vi "Load Settings from XML.vi"(8 "error in (no error)":errorcluster, 11 "Settings in":T1) -> (0 "error out":errorcluster, 3 "Settings out":T1)   [LabVIEW 2019, in "Settings.lvlib"]
doc: "Attempts to load previous user specified settings from an XML file.\n\nThis VI will not generate an error. If a suitable XML file can't be loaded and parsed then it will simply return the default settings."
uses:
  Settings.lvlib
  Settings.ctl
  Acquisition/Hardware Configuration.ctl
  Logging/Logging Configuration.ctl
  <vilib>/Utility/xml.llb/Read From XML File(string).vi
  <vilib>/Utility/xml.llb/Write to XML File(string).vi
  Acquisition/Acquisition.lvlib
  Logging/Logging.lvlib
panel:
  # "(Scroll up for Settings Controls)"
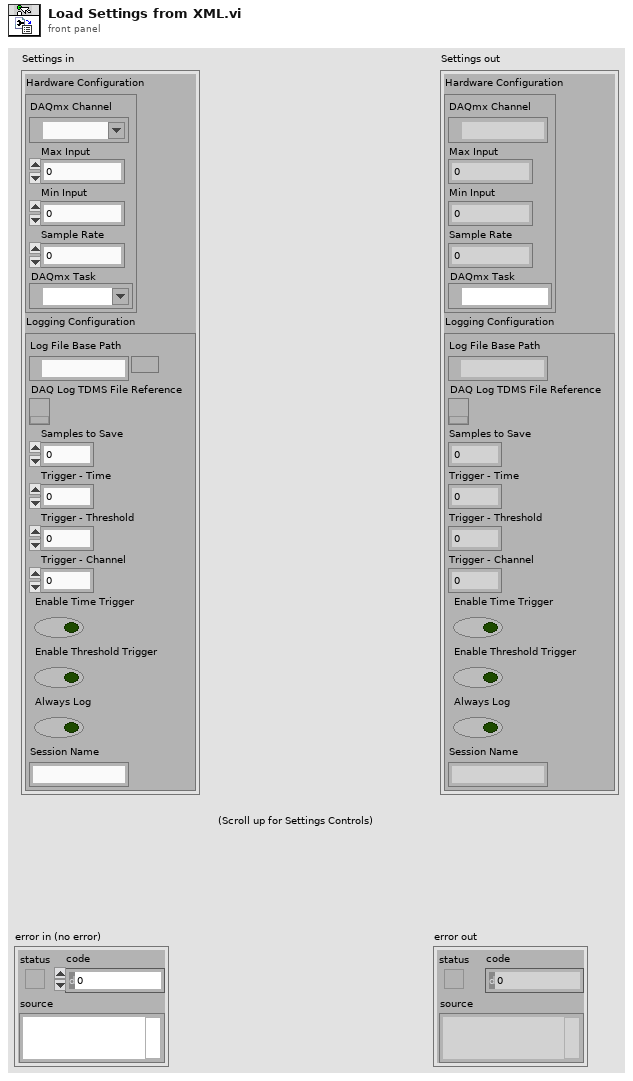
[diagram p1: front panel]
types:
  T1 = typedef "Settings.lvlib/Settings.ctl" = cluster{"Hardware Configuration":T2, "Logging Configuration":T3}
  T2 = typedef "Acquisition.lvlib/Hardware Configuration.ctl" = cluster{"DAQmx Channel":tag, "Max Input":dbl, "Min Input":dbl, "Sample Rate":dbl, "DAQmx Task":refnum<k21>}
  T3 = typedef "Logging.lvlib/Logging Configuration.ctl" = cluster{"Log File Base Path":path, "DAQ Log TDMS File Reference":refnum<k34>, "Samples to Save":u32, "Trigger - Time":u32, "Trigger - Threshold":dbl, "Trigger - Channel":u32, "Enable Time Trigger":bool, "Enable Threshold Trigger":bool, "Always Log":bool, "Session Name":string}
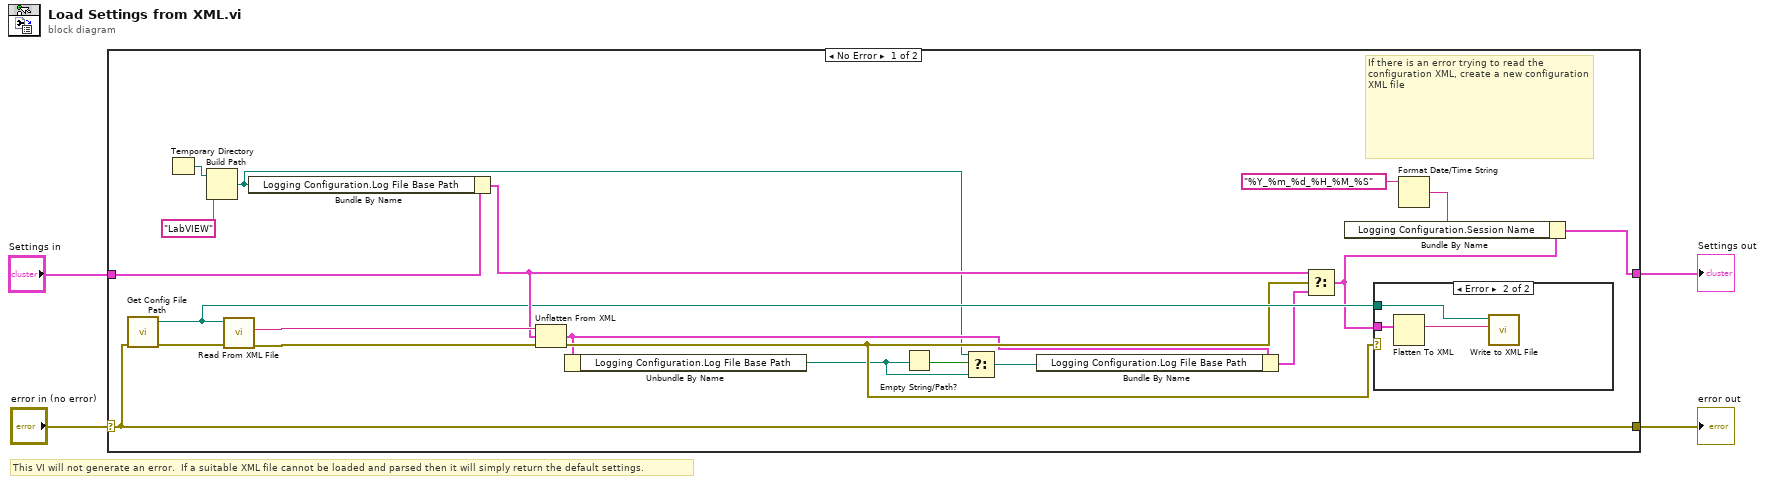
[diagram p0: block diagram]
diagram:
  # "This VI will not generate an error.  If a suitable XML file cannot be loaded and parsed then it will simply return the default settings."
  n1 = case shown="No Error" "error in (no error)" {
    selector: "error in (no error)" -> [w22 w29]
    tunnel: [w22 w29] -> w3
    tunnel: "Settings in" -> [w9 w28]
    tunnel: [w5 w28] -> w1
    frame No Error {
      # "If there is an error trying to read the configuration XML, create a new configuration XML file"
      n2 = call "Get Config File Path.vi"("error in (no error)"=w22) -> ("error out"=w24:errorcluster, "XML File Path"=w20:path)  [unwired: 9 in]
      n3 = Temporary Directory() -> (w12:path)
      n4 = Build Path(base path=w12, name or relative path="LabVIEW") -> (appended path=w10:path)
      n5 = call-poly <vilib>:"Read From XML File.vi"("error in (no error)"=w24, "XML File Path"=w20) -> ("error out"=w19:errorcluster, "XML Elements"=w23:string)  [unwired: 7 in, 1 out]
      n6 = Bundle By Name(cluster=w9, "Logging Configuration.Log File Base Path"=w10) -> (w21:T1)
      n7 = Unflatten From XML(xml string=w23, type=w21, error in (no error)=w19) -> (value=w15:T1, error out=w18:errorcluster)
      n8 = Unbundle By Name(w15) -> ("Logging Configuration.Log File Base Path"=w13:path)
      n9 = Empty String/Path?(string/path=w13) -> (empty?=w17:bool)
      n10 = Select(t=w10, s=w17, f=w13) -> (s? t:f=w16:path)
      n11 = Bundle By Name(cluster=w15, "Logging Configuration.Log File Base Path"=w16) -> (w14:T1)
      n12 = Select(t=w21, s=w18, f=w14) -> (s? t:f=w6:T1)
      n13 = case shown="Error" w18 {
        tunnel: w6 -> [_ w27]
        tunnel: w20 -> [_ w25]
        frame No Error {
        }
        frame Error {
          n14 = Flatten To XML(anything=w27) -> (xml string=w26:string)
          n15 = call-poly <vilib>:"Write to XML File.vi"("XML Input"=w26, "XML File Path"=w25) -> ()  [unwired: 7 in, 3 out]
        }
      }
      n16 = Format Date/Time String(time format string (%c)="%Y_%m_%d_%H_%M_%S") -> (date/time string=w7:string)  [unwired: 2 in]
      n17 = Bundle By Name(cluster=w6, "Logging Configuration.Session Name"=w7) -> (w5:T1)
    }
    frame Error {
    }
  }
  "error out" <- w3
  "Settings out" <- w1
